vi "Toggle Report Open Close.vi"(8 "error in (no error)":errorcluster, 10 "Open":bool, 11 "Report Generator in":refnum<class "Report Generator.lvclass">) -> (0 "error out":errorcluster, 3 "Report Generator out":refnum<class "Report Generator.lvclass">)   [LabVIEW 2023, in "Report Generator.lvlib" / "Report Generator.lvclass"]
doc: "This routine handles the data queue to close or open a report."
uses:
  Library/Report Generator.lvclass
  builds/Framework/Engine.lvlibp/Engine/Accessors/Read Report Q.vi
  builds/Tools/QDMH.lvlibp/Private/Enqueue Single State.vi
  builds/Tools/QDMH.lvlibp/Library/QDMH.lvclass
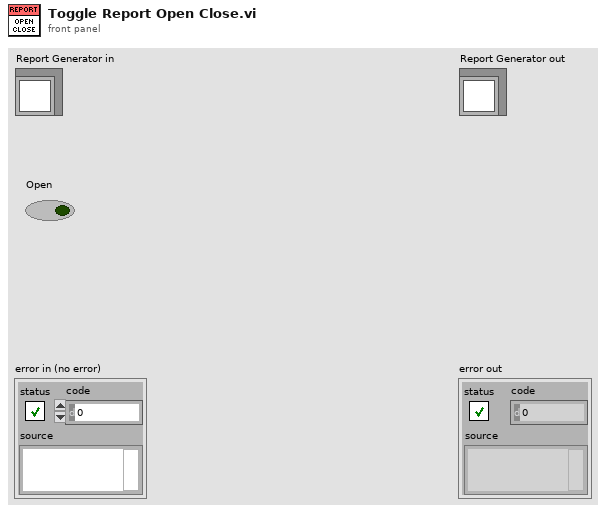
[diagram p1: front panel]
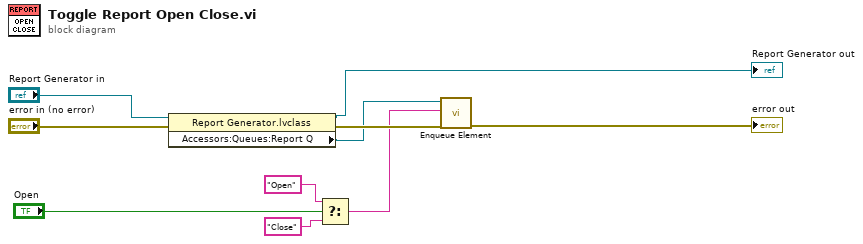
[diagram p0: block diagram]
diagram:
  n1 = property class="Report Generator.lvclass"(reference="Report Generator in", error in="error in (no error)") -> (reference out=→"Report Generator out":refnum<class "Report Generator.lvclass">, error out=w9:errorcluster, "Accessors:Queues:Report Q"=w8:refnum<class "QDMH.lvclass">)
  n2 = Select(t="Open", s="Open", f="Close") -> (s? t:f=w1:string)
  n3 = call-poly "Enqueue Element.vi"("error in (no error)"=w9, "String"=w1, "QDMH in"=w8) -> ("error out"=→"error out":errorcluster)  [unwired: 7 in, 1 out]
